vi "Measure DC offset.vi"(8 "Error In":errorcluster, 10 "Offset duration":dbl format="%0.2f", 11 "Waveform":waveform(dbl)) -> (0 "Error Out":errorcluster, 2 "Offset":dbl format="%0.2f")   [LabVIEW 2015]
uses:
  <vilib>/Waveform/WDTOps.llb/WDT Get Waveform Subset DBL.vi
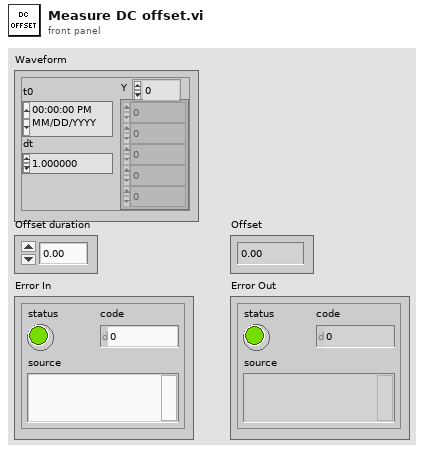
[diagram p1: front panel]
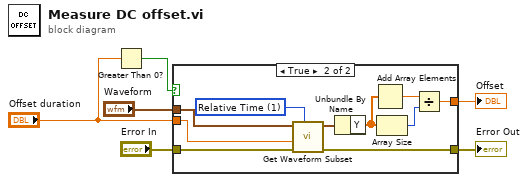
[diagram p0: block diagram]
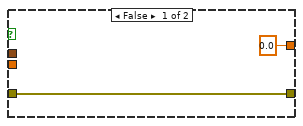
[diagram p2: hidden frame]
diagram:
  n1 = Greater Than 0?(x="Offset duration") -> (x > 0?=w3:bool)
  n2 = case shown="True" w3 {
    tunnel: "Offset duration" -> [_ w13]
    tunnel: "Waveform" -> [_ w12]
    tunnel: "Error In" -> [w8 w11]
    tunnel: [w8 w10] -> w2
    tunnel: [0.0 w9] -> w1
    frame False {
    }
    frame True {
      w18 = u16 1 items=["Index", "Relative Time"] ("start/duration format")
      n3 = call-poly <vilib>:"Get Waveform Subset.vi"("start/duration format"=w18, "error in (no error)"=w11, "duration"=w13, "waveform in"=w12) -> ("error out"=w10:errorcluster, "waveform out"=w14:waveform(dbl))  [unwired: 1 in, 3 out]
      n4 = Unbundle By Name(w14) -> ("Y"=w16:dbl[])
      n5 = Add Array Elements(numeric array=w16) -> (sum=w15:dbl)
      n6 = Array Size(array=w16) -> (size(s)=w17:i32)
      n7 = Divide(x=w15, y=w17) -> (x/y=w9:dbl)
    }
  }
  "Error Out" <- w2
  "Offset" <- w1
